vi "_SendCommand.vi"(8 "error in":errorcluster, 10 "Command":string, 11 "Instrument Channel":string="GPIB/0:4,0") -> (0 "error out":errorcluster, 3 "Instrument Channel out":string="GPIB/0:4,0")   [LabVIEW 2020, in "FCR100.lvlib"]
doc: "Send command string to instrument channel."
uses:
  FCR100.lvlib
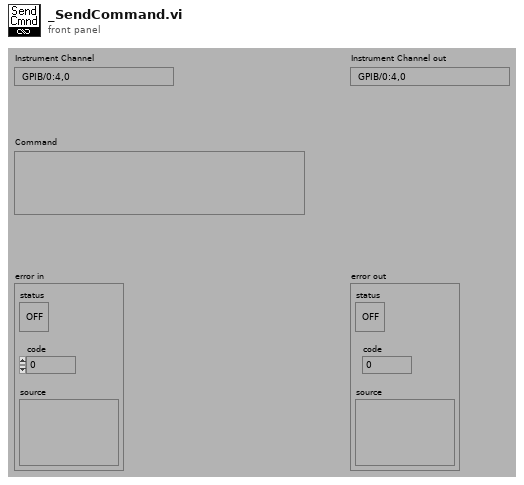
[diagram p1: front panel]
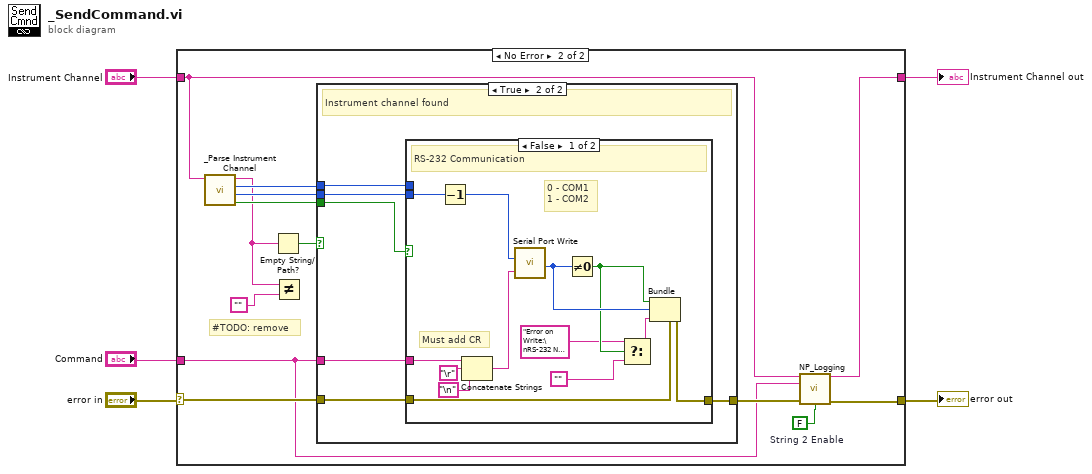
[diagram p0: block diagram]
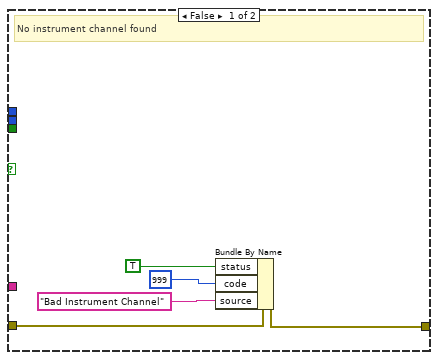
[diagram p3: hidden frame]
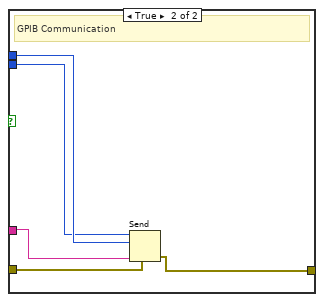
[diagram p4: hidden frame]
diagram:
  n1 = case shown="No Error" "error in" {
    selector: "error in" -> [w6 w20]
    tunnel: "Instrument Channel" -> [w7 w10]
    tunnel: [w7 w9] -> w3
    tunnel: [w6 w11] -> w2
    tunnel: "Command" -> [_ w8]
    frame Error {
      # "Error Status is True"
    }
    frame No Error {
      w13 = FALSE  # String 2 Enable
      # "#TODO: remove"
      n2 = call "_Parse Instrument Channel.vi"("Instrument Channel"=w10) -> ("T - GPIB, F - RS232"=w17:bool, "Hardware Address"=w16:i32, "Instrument Address"=w18:i16, "Instrument Channel out"=w15:string)  [unwired: 6 in, 1 out]
      n3 = Empty String/Path?(string/path=w15) -> (empty?=w14:bool)
      n4 = Not Equal?(x=w15, y="") -> ()  [unwired: 1 out]
      n5 = case shown="True" w14 {
        tunnel: w20 -> [w22 w31]
        tunnel: [w21 w30] -> w12
        tunnel: w18 -> [_ w29]
        tunnel: w17 -> [_ w28]
        tunnel: w16 -> [_ w27]
        tunnel: w8 -> [_ w26]
        frame False {
          # "No instrument channel found"
          n6 = Bundle By Name(cluster=w22, "status"=TRUE, "code"=999, "source"="Bad Instrument Channel") -> (w21:errorcluster)
        }
        frame True {
          # "Instrument channel found"
          n7 = case shown="False" w28 {
            tunnel: w26 -> [w44 w49]
            tunnel: w31 -> [w43 w48]
            tunnel: [w42 w47] -> w30
            tunnel: w29 -> [_ w46]
            tunnel: w27 -> [w32 w45]
            frame False {
              # "0 - COM1\n1 - COM2"
              # "Must add CR"
              # "RS-232 Communication"
              n8 = Decrement(x=w32) -> (x-1=w33:i32)
              n9 = Concatenate Strings(w44, "\r", "\n") -> (w37:string)
              n10 = call <vilib>:"Serial Port Write.vi"("string to write"=w37, "port number"=w33) -> ("error code"=w41:i32)
              n11 = Not Equal To 0?(x=w41) -> (x != 0?=w40:bool)
              n12 = Select(t="Error on Write:\nRS-232 Not available.", s=w40, f="") -> (s? t:f=w39:string)
              n13 = Bundle(cluster=w43, "status"=w40, "code"=w41, "source"=w39) -> (w42:errorcluster)
            }
            frame True {
              # "GPIB Communication"
              n14 = Send(0:w45, 2:w46, 4:w48, 5:w49) -> (8:w47:errorcluster)  [unwired: 1 in, 2 out]
            }
          }
        }
      }
      n15 = call "NP_Logging.vi"("Instrument Channel"=w10, "String 1 {Write} (in)"=w8, "error in (no error)"=w12, "String 2 Enable (T)"=w13) -> ("Instrument Channel out"=w9:string, "error out"=w11:errorcluster)  [unwired: 8 in, 2 out]
    }
  }
  "Instrument Channel out" <- w3
  "error out" <- w2
